vi "Remove from Query.vi"(8 "error in (no error)":errorcluster, 10 "key":string, 11 "URI in":refnum<class "URI.lvclass">) -> (0 "error out":errorcluster, 1 "deleted":bool, 3 "URI out":refnum<class "URI.lvclass">)   [LabVIEW 2013, in "openURI.lvlib" / "URI.lvclass"]
uses:
  URI.lvclass
  URI.lvclass/URI.ctl
  components/query/URI-Component.Query.lvclass/URI-Component.Query.ctl
  components/query/URI-Component.Query.lvclass
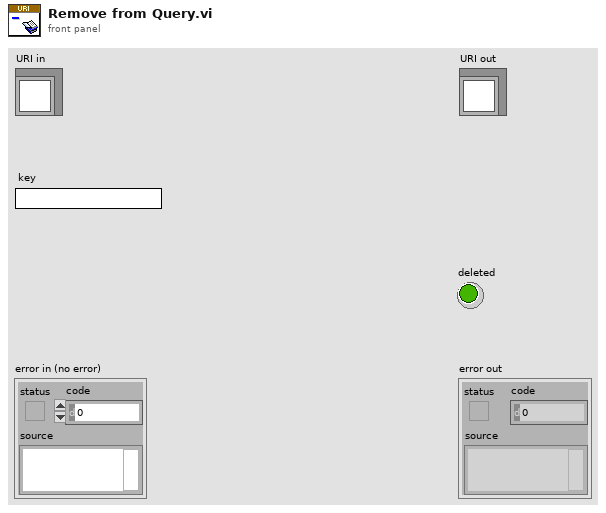
[diagram p1: front panel]
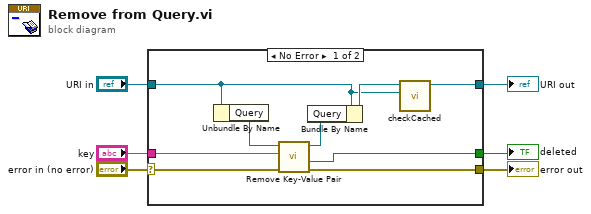
[diagram p0: block diagram]
diagram:
  n1 = case shown="No Error" "error in (no error)" {
    selector: "error in (no error)" -> [w10 w17]
    tunnel: [w11 w17] -> w5
    tunnel: [w8 w16] -> w3
    tunnel: "URI in" -> [w7 w16]
    tunnel: "key" -> [w13 _]
    tunnel: [w12 _] -> w1
    frame No Error {
      n2 = Unbundle By Name(w7) -> ("Query"=w15:refnum<class "URI-Component.Query.lvclass">)
      n3 = call "Remove Key-Value Pair.vi"("error in (no error)"=w10, "key"=w13, "URI-Component.Query in"=w15) -> ("error out"=w11:errorcluster, "deleted"=w12:bool, "URI-Component.Query"=w14:refnum<class "URI-Component.Query.lvclass">)  [unwired: 6 in]
      n4 = Bundle By Name(cluster=w7, "Query"=w14) -> (w9:refnum<class "URI.lvclass">)
      n5 = call "checkCached.vi"("Old"=w7, "New URI"=w9) -> ("URI"=w8:refnum<class "URI.lvclass">)  [unwired: 9 in]
    }
    frame Error {
    }
  }
  "error out" <- w5
  "URI out" <- w3
  "deleted" <- w1
